vi "User Console Main.vi"(8 "error in (no error)":errorcluster) -> (0 "error out":errorcluster)   [LabVIEW 2020, in "User Console.lvlib"]
doc: "This is the Main VI for the User Console Module."
uses:
  User Console.lvlib
  Private Controls/Transactions.ctl
  Private Controls/Keypad.ctl
  Private Controls/FG Actions.ctl
  Private Controls/Module Data.ctl
  Private Controls/Message Cluster.ctl
  Private Controls/Message enum.ctl
panel:
  in  "Card Reader":bool
  in  "Keypad":T1
  in  "Transactions":T2
  # "[Covers: UI2]"
  # "[Covers: UI2B]"
  # "[Covers: UI2A]"
  # "[Covers: UI2C]"
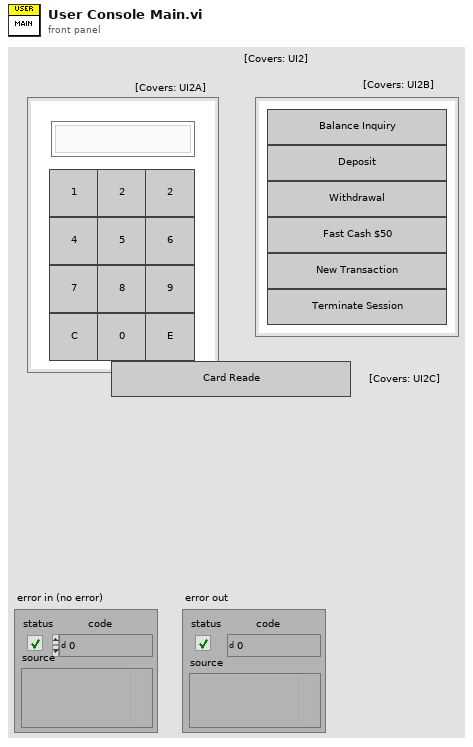
[diagram p1: front panel]
types:
  T1 = typedef "User Console.lvlib/Keypad.ctl" = cluster{"1":bool, "2":bool, "3":bool, "4":bool, "5":bool, "6":bool, "7":bool, "8":bool, "9":bool, "C":bool, "0":bool, "E":bool, "Screen":string}
  T2 = typedef "User Console.lvlib/Transactions.ctl" = cluster{"Balance Inquiry":bool, "Deposti":bool, "Withdrawal":bool, "Fast Cash":bool, "New Transaction":bool, "Terminate":bool}
  T3 = typedef "User Console.lvlib/Module Data.ctl" = cluster{"Data":variant}
  T4 = typedef "User Console.lvlib/FG Actions.ctl" = enum16{"Get", "Set", "Clear"}
  T5 = typedef "User Console.lvlib/Message Cluster.ctl" = cluster{"Message":T6, "Data":variant}
  T6 = typedef "User Console.lvlib/Message enum.ctl" = enum16{"Initialize", "State", "Error", "Exit"}
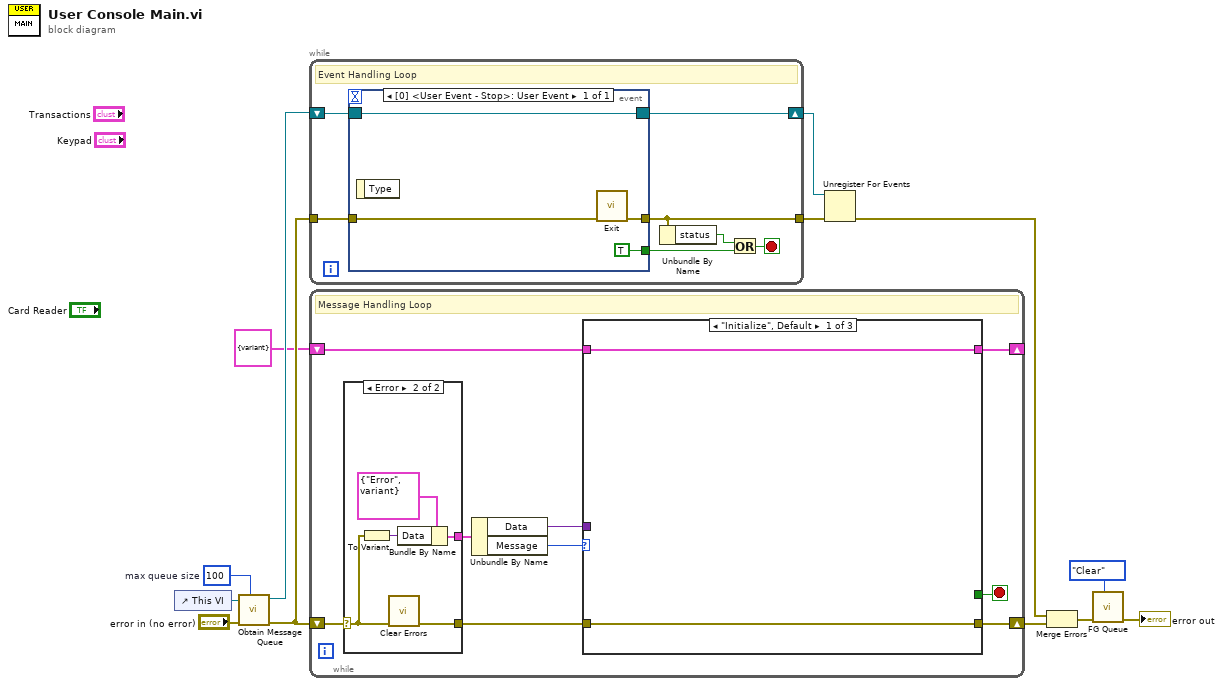
[diagram p0: block diagram]
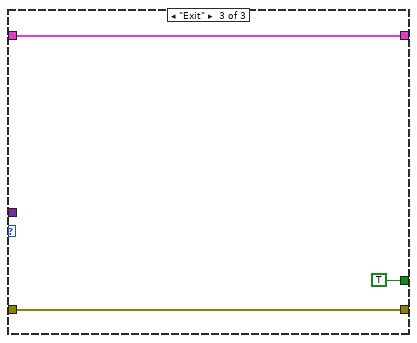
[diagram p3: hidden frame]
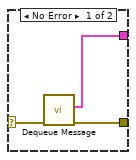
[diagram p4: hidden frame]
diagram:
  w7 = 100  # max queue size
  n1 = control-ref of="This VI"() -> (w8:refnum<vi>)
  n2 = call "Obtain Message Queue.vi"("max queue size (-1, unlimited)"=w7, "error in (no error)"="error in (no error)", "VI Reference"=w8) -> ("error out"=w3:errorcluster, "Event Registration Refnum"=w10:refnum<event-registration>)  [unwired: 7 in]
  n3 = while {
    shift-right: [w19] -> w11
    shift-left: w10 -> [w20]
    tunnel: w3 -> [w17]
    tunnel: [w15] -> w2
    stop <- w16 stop-if-true
    # "Event Handling Loop"
    n4 = event shown="[0] <User Event - Stop>: User Event" {
      selector: w20 -> [w21]
      dyn-events: [w21] -> w19
      timeout: _ -> [_]
      tunnel: [TRUE ("Discard?")] -> w18
      tunnel: w17 -> [w23]
      tunnel: [w22] -> w15
      event User Event {
        n5 = event-data() -> ()  [unwired: 1 in, 1 out]
        n6 = call "Exit.vi"("error in (no error)"=w23) -> ("error out"=w22:errorcluster)  [unwired: 10 in]
      }
    }
    n7 = Unbundle By Name(w15) -> ("status"=w14:bool)
    n8 = Or(x=w14, y=w18) -> (x .or. y?=w16:bool)
  }
  n9 = while {
    shift-right: [w28] -> w13
    shift-left: w3 -> [w33]
    shift-right: [w25] -> _
    shift-left: T3 {"Data"=variant} ("Message Cluster") -> [w26]
    stop <- w27 stop-if-true
    # "Message Handling Loop"
    n10 = case shown="Error" w33 {
      selector: w33 -> [w41 w47]
      tunnel: [w42 w48] -> w29
      tunnel: [w43 w44] -> w32
      frame No Error {
        n11 = call "Dequeue Message.vi"("error in (no error)"=w41) -> ("error out"=w42:errorcluster, "Element"=w43:T5)  [unwired: 9 in]
      }
      frame Error {
        n12 = To Variant(anything=w47) -> (Variant=w45:variant)
        n13 = call <vilib>:"Clear Errors.vi"("error in (no error)"=w47) -> ("error out"=w48:errorcluster)  [unwired: 5 in, 1 out]
        n14 = Bundle By Name(cluster=T5 {"Message"=enum."Error", "Data"=variant} ("Message Cluster"), "Data"=w45) -> (w44:T5)
      }
    }
    n15 = Unbundle By Name(w32) -> ("Data"=w30:variant, "Message"=w31:T6)
    n16 = case shown="\"Initialize\", Default" w31 {
      tunnel: w30 -> [_ _ _]
      tunnel: w29 -> [w35 w37 w40]
      tunnel: [w35 w37 w40] -> w28
      tunnel: [_ _ TRUE] -> w27
      tunnel: w26 -> [w34 w36 w38]
      tunnel: [w34 w36 w38] -> w25
      frame "Initialize", Default {
      }
      frame "Error" {
      }
      frame "Exit" {
      }
    }
  }
  n17 = Unregister For Events(event registration refnum=w11, error in=w2) -> (error out=w12:errorcluster)
  n18 = Merge Errors(w12, w13) -> (w5:errorcluster)
  n19 = call "FG Queue.vi"("FG Actions"=FG_Actions."Clear", "error in (no error)"=w5) -> ("error out"=→"error out":errorcluster)  [unwired: 8 in, 1 out]
